vi "Add On Event Message.vi"(8 "error in (no error)":errorcluster, 9 "Message To Send":T1, 10 "Event":string, 11 "Observable Actor in":refnum<class "Observable Actor.lvclass">) -> (0 "error out":errorcluster, 3 "Observable Actor out":refnum<class "Observable Actor.lvclass">)   [LabVIEW 2014, in "Observable Actor.lvlib" / "Observable Actor.lvclass"]
uses:
  Observable Actor.lvclass
  Model/Data/MessageToSend.ctl
  <vilib>/ActorFramework/Message Enqueuer/Message Enqueuer.lvclass
  <vilib>/ActorFramework/Message/Message.lvclass
  Observable Actor.lvclass/Observable Actor.ctl
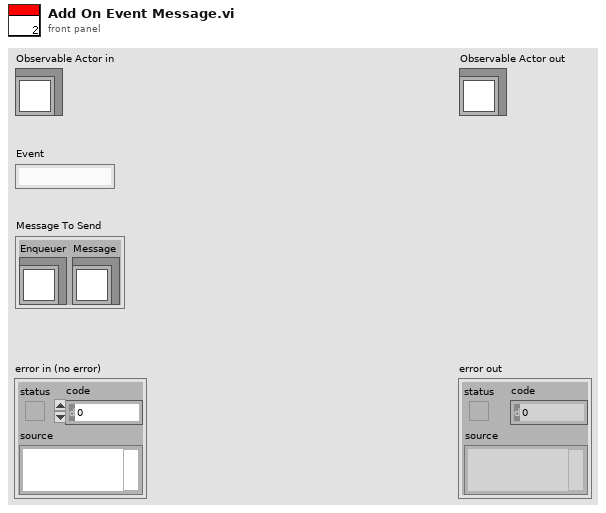
[diagram p1: front panel]
types:
  T1 = typedef "MessageToSend.ctl" = cluster{"Enqueuer":refnum<class "Message Enqueuer.lvclass">, "Message":refnum<class "Message.lvclass">}
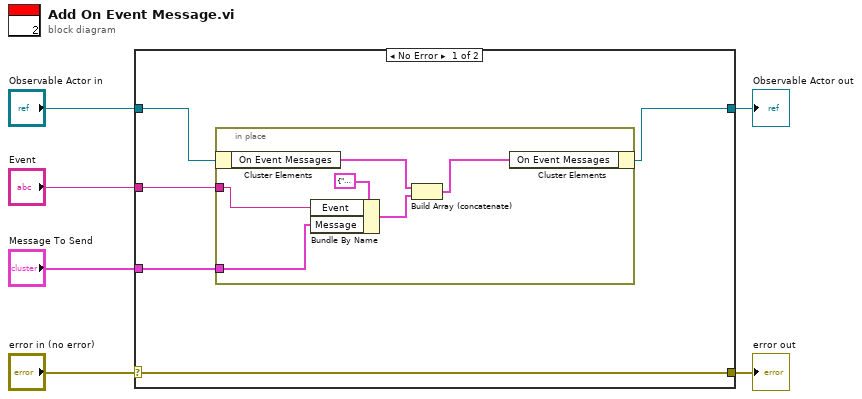
[diagram p0: block diagram]
diagram:
  n1 = case shown="No Error" "error in (no error)" {
    selector: "error in (no error)" -> [w11 w19]
    tunnel: [w11 w19] -> w5
    tunnel: [w9 w18] -> w3
    tunnel: "Observable Actor in" -> [w10 w18]
    tunnel: "Message To Send" -> [w7 _]
    tunnel: "Event" -> [w8 _]
    frame No Error {
      n2 = in-place {
        in-place-border: w8 -> [w14]
        in-place-border: w7 -> [w13]
        n3 = in-place-cluster #1(w10) -> ("On Event Messages"=w16:cluster{"Event":string, "Message To Send":T1}[])
        n4 = Bundle By Name(cluster=cluster{"Event":string, "Message":T1} {"Event"="", "Message"={"Enqueuer"=refnum, "Message"=refnum}} ("element"), "Event"=w14, "Message"=w13) -> (w12:cluster{"Event":string, "Message":T1})
        n5 = Build Array (concatenate)(w16, w12) -> (w17:cluster{"Event":string, "Message":T1}[])
        n6 = in-place-cluster #1("On Event Messages"=w17) -> (w9:refnum<class "Observable Actor.lvclass">)
      }
    }
    frame Error {
    }
  }
  "error out" <- w5
  "Observable Actor out" <- w3
